vi "RichToFlatrfcontrol_NMapRequest.vi"(5 "OutputClusterType":T1, 11 "InputCluster":T2) -> (3 "OutputCluster":T1)   [LabVIEW 2024, in "FlexSDR_gRPC_client.lvlib"]
uses:
  FlexSDR_gRPC_client.lvlib
  rfcontrol_NMapRequest.ctl
  rfcontrol_NMapRequest_Flat.ctl
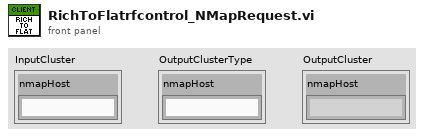
[diagram p1: front panel]
types:
  T1 = typedef "FlexSDR_gRPC_client.lvlib/rfcontrol_NMapRequest_Flat.ctl" = cluster{"nmapHost":string}
  T2 = typedef "FlexSDR_gRPC_client.lvlib/rfcontrol_NMapRequest.ctl" = cluster{"nmapHost":string}
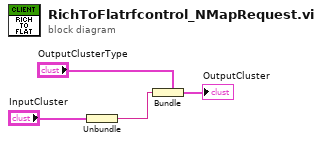
[diagram p0: block diagram]
diagram:
  n1 = Unbundle "Unbundle"("InputCluster") -> ("nmapHost"=w1:string)
  n2 = Bundle "Bundle"(cluster="OutputClusterType", "nmapHost"=w1) -> (→"OutputCluster":T1)
